vi "geterror.vi"(8 "error in (no error)":errorcluster, 11 "MSCU":refnum<class "MSCU.lvclass">) -> (0 "error out":errorcluster, 2 "Error":string, 3 "MSCU":refnum<class "MSCU.lvclass">)   [LabVIEW 2019, in "MSCU.lvclass"]
uses:
  MSCU.lvclass
  MSCU.lvclass/MSCU.ctl
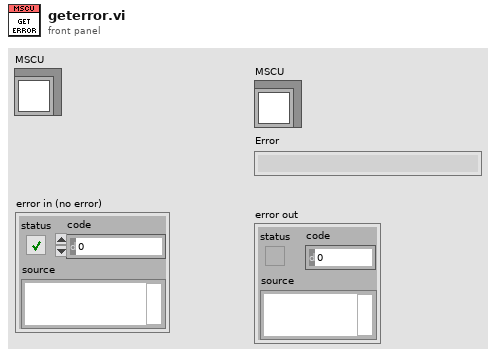
[diagram p1: front panel]
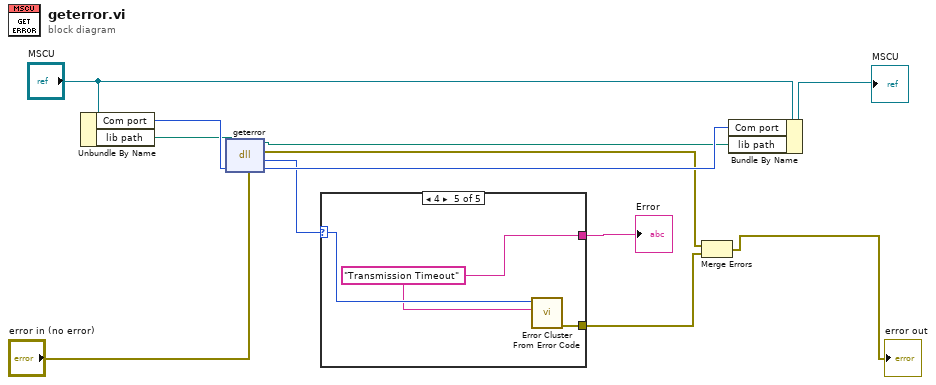
[diagram p0: block diagram]
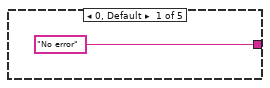
[diagram p2: hidden frame]
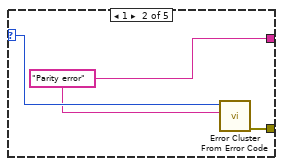
[diagram p3: hidden frame]
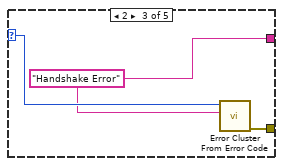
[diagram p4: hidden frame]
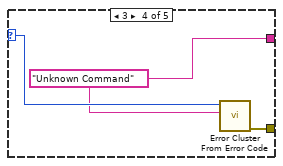
[diagram p5: hidden frame]
diagram:
  n1 = Unbundle By Name("MSCU") -> ("Com port"=w5:i32, "lib path"=w4:path)
  n2 = dll-call lib="C:/Program Files (x86)/Nanonis/SPM Controller/data/MSCU.dll" fn="geterror"(path in=w4, error in="error in (no error)", "Comport"=w5) -> (path out=w2:path, error out=w10:errorcluster, "return type"=w8:i32, "Comport"=w11:i32)  [unwired: 1 in]
  n3 = case shown="4" w8 {
    selector: w8 -> [_ w16 w19 w22 w25]
    tunnel: ["No error" w14 w17 w20 w23] -> w9
    tunnel: [_ w15 w18 w21 w24] -> w12
    frame 0, Default {
    }
    frame 1 {
      w14 = "Parity error"
      n4 = call <vilib>:"Error Cluster From Error Code.vi"("error message (\"\")"=w14, "error code (0)"=w16) -> ("error out"=w15:errorcluster)  [unwired: 7 in]
    }
    frame 2 {
      w17 = "Handshake Error"
      n5 = call <vilib>:"Error Cluster From Error Code.vi"("error message (\"\")"=w17, "error code (0)"=w19) -> ("error out"=w18:errorcluster)  [unwired: 7 in]
    }
    frame 3 {
      w20 = "Unknown Command"
      n6 = call <vilib>:"Error Cluster From Error Code.vi"("error message (\"\")"=w20, "error code (0)"=w22) -> ("error out"=w21:errorcluster)  [unwired: 7 in]
    }
    frame 4 {
      w23 = "Transmission Timeout"
      n7 = call <vilib>:"Error Cluster From Error Code.vi"("error message (\"\")"=w23, "error code (0)"=w25) -> ("error out"=w24:errorcluster)  [unwired: 7 in]
    }
  }
  "Error" <- w9
  n8 = Merge Errors(w10, w12) -> (→"error out":errorcluster)
  n9 = Bundle By Name(cluster="MSCU", "Com port"=w11, "lib path"=w2) -> (→"MSCU":refnum<class "MSCU.lvclass">)
